vi "counter.vi"   [LabVIEW 2015]
uses:
  <vilib>/DAQmx/create/channels.llb/DAQmx Create Channel (CI-Count Edges).vi
  <resource>/objmgr/daqmx.rc
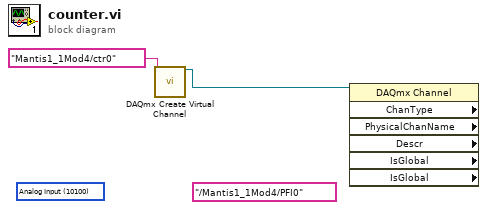
[diagram p0: block diagram]
diagram:
  (unwired) 10100 items=["Analog Input"=10100, "Analog Output"=10102, "Digital Input"=10151, "Digital Output"=10153, "Counter Input"=10131, "Counter Output"=10132] ("ChanType")
  (unwired) tag "/Mantis1_1Mod4/PFI0" ("CI.CtrTimebaseSrc")
  n1 = call-poly <vilib>:"DAQmx Create Virtual Channel.vi"("counter"=tag "Mantis1_1Mod4/ctr0") -> ("task out"=w1:refnum<k21>)  [unwired: 13 in, 1 out]
  n2 = property class="DAQmx Channel" props=["ChanType", "PhysicalChanName", "Descr", "IsGlobal", "IsGlobal"](reference=w1) -> ()  [unwired: 1 in, 7 out]
